vi "Help2--Const.vi"() -> (3 "Help2 Command":string)   [LabVIEW 2017, in "Communications Library.lvlib"]
uses:
  Communications Library.lvlib
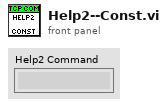
[diagram p1: front panel]
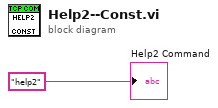
[diagram p0: block diagram]
diagram:
  "Help2 Command" <- "help2" ("data in")
